vi "Process Verification Response.vi"(8 "error in":errorcluster, 10 "serverHash":u8[](array[numeric]), 11 "srp":T1) -> (0 "error out":errorcluster, 3 "srp":T1)   [LabVIEW 2016, in "SRP.lvlib"]
uses:
  <vilib>/addons/InsightCM/SRP/SRP.lvlib
  <vilib>/addons/InsightCM/SRP/controls/DVR_data.ctl
  <vilib>/addons/InsightCM/SRP/controls/data.ctl
  <vilib>/addons/InsightCM/SRP/libraries/win32Urelease/brsrp.dll
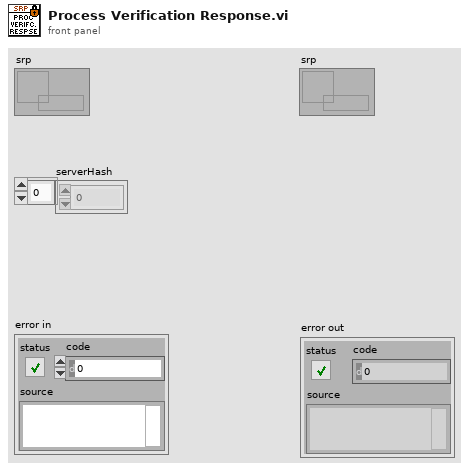
[diagram p1: front panel]
types:
  T1 = typedef "SRP.lvlib/DVR_data.ctl" = refnum<data-value>
  T2 = typedef "SRP.lvlib/data.ctl" = cluster{"SessionKey":u8[], "ClientHash":u8[], "PublicKeyA":u8[], "PrivateKeyA":u8[]}
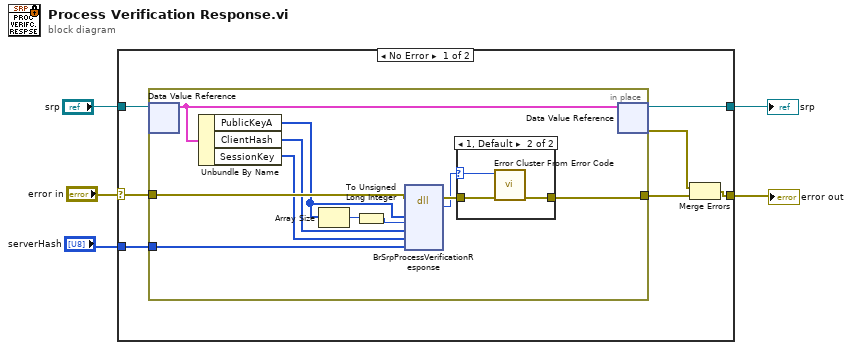
[diagram p0: block diagram]
diagram:
  n1 = case shown="No Error" "error in" {
    selector: "error in" -> [w11 w29]
    tunnel: [w7 w29] -> w5
    tunnel: "srp" -> [w10 w28]
    tunnel: [w9 w28] -> w2
    tunnel: "serverHash" -> [w8 _]
    frame No Error {
      n2 = in-place {
        in-place-border: [w22] -> w12
        in-place-border: w11 -> [w20]
        in-place-border: w8 -> [w16]
        n3 = in-place-dvr #1(w10) -> (w17:T2)  [unwired: 1 out]
        n4 = Unbundle By Name(w17) -> ("PublicKeyA"=w13:u8[], "ClientHash"=w19:u8[], "SessionKey"=w18:u8[])
        n5 = Array Size(array=w13) -> (size(s)=w15:i32)
        n6 = To Unsigned Long Integer(number=w15) -> (unsigned 32bit integer=w14:u32)
        n7 = dll-call lib="C:/Program Files (x86)/National Instruments/LabVIEW 2016/vi.lib/addons/InsightCM/SRP/libraries/win32Urelease/brsrp.*" fn="BrSrpProcessVerificationResponse"(error in=w20, "publicKeyA"=w13, "publicKeyA_length"=w14, "clientHash"=w19, "sessionKey"=w18, "serverHash"=w16) -> (error out=w23:errorcluster, "return type"=w21:i32)  [unwired: 7 in, 1 out]
        n8 = case shown="1, Default" w21 {
          selector: w21 -> [_ w25]
          tunnel: w23 -> [w24 w27]
          tunnel: [w24 w26] -> w22
          frame 0 {
          }
          frame 1, Default {
            n9 = call <vilib>:"Error Cluster From Error Code.vi"("error in (no error)"=w27, "error code (0)"=w25) -> ("error out"=w26:errorcluster)  [unwired: 7 in]
          }
        }
        n10 = in-place-dvr #1(w17) -> (w9:T1, w6:errorcluster)
      }
      n11 = Merge Errors(w6, w12) -> (w7:errorcluster)
    }
    frame Error {
    }
  }
  "error out" <- w5
  "srp" <- w2
